vi "captureAverage_v23-malusBook.vi"(8 "Numeric":i32, 10 "Image In":T2, 11 "Session In":T1) -> (2 "Image Out":T2)   [LabVIEW 2022 SP3]
uses:
  <vilib>/vision/Image Controls.llb/IMAQ Image.ctl
  <vilib>/userdefined/High Color/IMAQdx.ctl
  <vilib>/vision/driver/NI_Vision_Acquisition_Software.lvlib
panel:
  out "x+y":sgl[][](array[numeric])
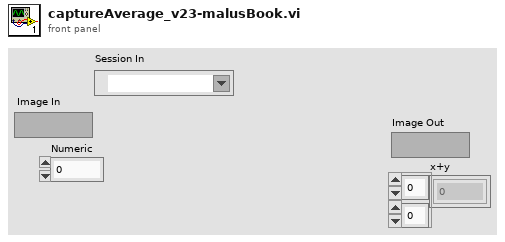
[diagram p1: front panel]
types:
  T1 = typedef "IMAQdx.ctl" = refnum<k21>
  T2 = typedef "IMAQ Image.ctl" = refnum<image>
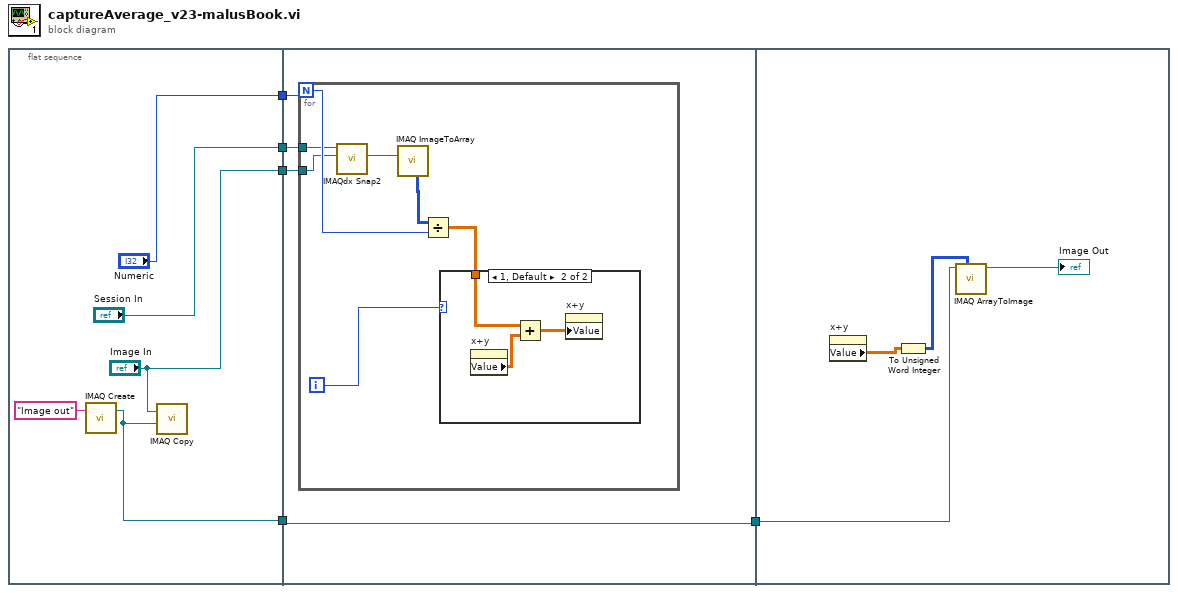
[diagram p0: block diagram]
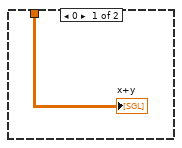
[diagram p2: hidden frame]
diagram:
  n1 = flat-sequence {
    tunnel: ["Numeric"] -> w5
    tunnel: ["Image In"] -> w4
    tunnel: ["Session In"] -> w3
    tunnel: [w8] -> w1
    tunnel: w5 -> [w14]
    tunnel: w4 -> [w13]
    tunnel: w3 -> [w12]
    tunnel: [w11] -> w2
    tunnel: w1 -> [w11]
    tunnel: w2 -> [w26]
    frame #0 {
      n2 = call "IMAQ Create"("Image Name"="Image out") -> ("New Image"=w8:T2)  [unwired: 4 in, 1 out]
      n3 = call "IMAQ Copy"("Image Dst"=w8, "Image Src"="Image In") -> ()  [unwired: 4 in, 2 out]
    }
    frame #1 {
      n4 = for {
        N: w14 -> [w19]
        tunnel: w13 -> [w16]
        tunnel: w12 -> [w17]
        i -> [w21]
        n5 = call <vilib>:"IMAQdx Snap2.vi"("Image In"=w16, "Session In"=w17) -> ("Image Out"=w15:T2)  [unwired: 7 in, 2 out]
        n6 = call "IMAQ ImageToArray"("Image"=w15) -> ("Image Pixels (U16)"=w20:u16[][])  [unwired: 3 in, 4 out]
        n7 = Divide(x=w20, y=w19) -> (x/y=w18:dbl[][])
        n8 = case shown="1, Default" w21 {
          tunnel: w18 -> [w22 w25]
          frame 0 {
            "x+y" <- w22
          }
          frame 1, Default {
            n9 = property on="x+y" class="Arr (strict)"() -> ("Value"=w24:sgl[][])  [unwired: 2 in, 2 out]
            n10 = Add(x=w25, y=w24) -> (x+y=w23:dbl[][])
            n11 = property on="x+y" class="Arr (strict)"("Value"=w23) -> ()  [unwired: 2 in, 2 out]
          }
        }
      }
    }
    frame #2 {
      n12 = property on="x+y" class="Arr (strict)"() -> ("Value"=w29:sgl[][])  [unwired: 2 in, 2 out]
      n13 = To Unsigned Word Integer(number=w29) -> (unsigned 16bit integer=w28:u16[][])
      n14 = call "IMAQ ArrayToImage"("Image Pixels (U16)"=w28, "Image"=w26) -> ("Image Out"=→"Image Out":T2)  [unwired: 8 in, 1 out]
    }
  }
